vi "100kHz PID - Arbitration.vi"() -> ()   [LabVIEW 2010]
uses:
  <vilib>/eio/EIONode/EIONode.xnode
  <vilib>/rvi/eio/nirviEIOImplementation/nirviEIOImplementation.xnode
  <vilib>/rvi/eio/common/nirviEmuClasses.ctl
  <vilib>/addons/control/pid/fpga.llb/XNode/niFpgaPID.xnode
  <vilib>/rvi/eio/common/nirviEmuTemplateMethod_noerrors.vi
panel:
  in  "PID.Setpoint.PID 3":i16
  in  "PID.Proportional Gain.PID 3":i16=1
  in  "PID.Integral Gain.PID 3":i16
  in  "PID.Derivative Gain.PID 3":i16
  out "PID.Num Ticks 3":u32
  in  "PID.Setpoint.PID 2":i16
  in  "PID.Proportional Gain.PID 2":i16=1
  in  "PID.Integral Gain.PID 2":i16
  in  "PID.Derivative Gain.PID 2":i16
  out "PID.Num Ticks2":u32
  out "PID.Num Ticks 1":u32
  out "PID.Num Ticks":u32
  in  "PID.Setpoint.PID 1":i16
  in  "PID.Proportional Gain.PID 1":i16=1
  in  "PID.Integral Gain.PID 1":i16
  in  "PID.Derivative Gain.PID 1":i16
  in  "PID.Setpoint.PID 0":i16
  in  "PID.Proportional Gain.PID 0":i16=1
  in  "PID.Integral Gain.PID 0":i16
  in  "PID.Derivative Gain.PID 0":i16
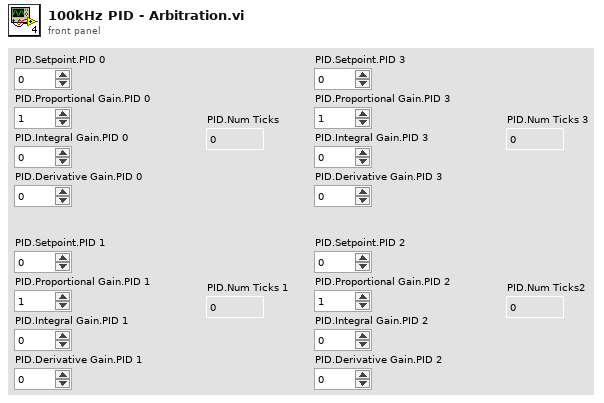
[diagram p1: front panel]
types:
  T1 = cluster{"proportional gain (Kc)":i16, "integral gain (Kc*Ts/Ti)":i16, "derivative gain (Kc*Td/Ts)":i16}
  T2 = typedef "nirviEmuClasses.ctl" = enum16{"IO Read", "IO Write", "Method", "Property Read", "Property Write"}
  T3 = cluster{"proportional gain (Kc)":fxp<+/-,16,8>, "proportional gain (Kc)":fxp<+/-,16,8>, "proportional gain (Kc)":fxp<+/-,16,8>}
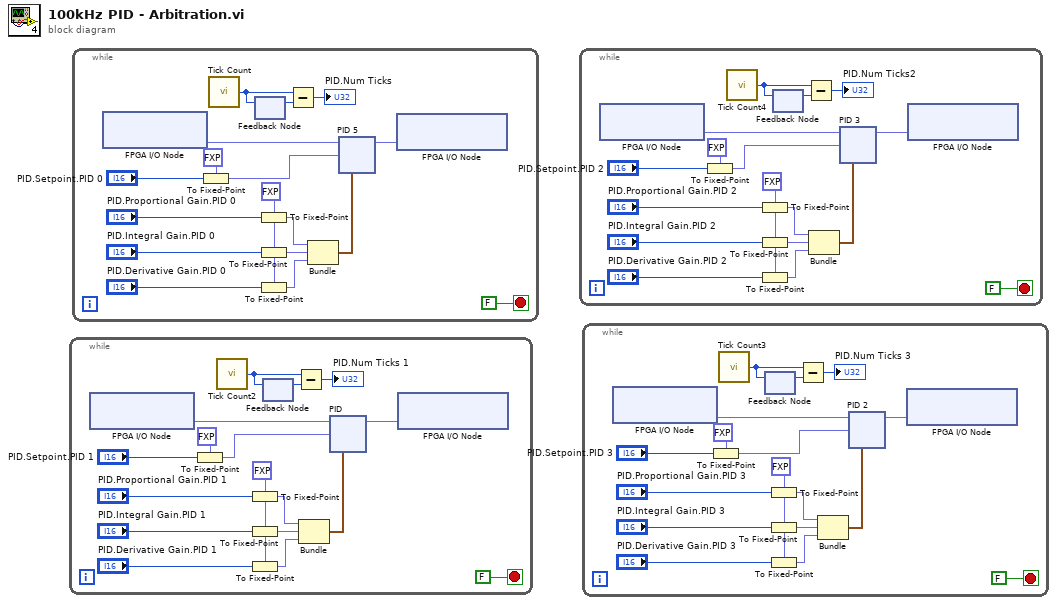
[diagram p0: block diagram]
diagram:
  n1 = while {
    stop <- FALSE stop-if-true
    w10 = fxp<+/-,16,8> 0.0 ("proportional gain (Kc)")
    n2 = xnode "FPGA I/O Node"() -> ("NI 9215/AI1"=w6:fxp<+/-,20,5>)  [unwired: 1 in, 1 out]
    n3 = To Fixed-Point(fixed-point type=fxp<+/-,16,5> 0.0 ("setpoint"), number="PID.Setpoint.PID 1") -> (fixed-point=w8:fxp<+/-,16,5>)
    n4 = call "Tick Count2"() -> ("Tick Count(Ticks)"=w2:u32)
    n5 = To Fixed-Point(fixed-point type=w10, number="PID.Proportional Gain.PID 1") -> (fixed-point=w13:fxp<+/-,16,8>)
    n6 = To Fixed-Point(fixed-point type=w10, number="PID.Integral Gain.PID 1") -> (fixed-point=w12:fxp<+/-,16,8>)
    n7 = To Fixed-Point(fixed-point type=w10, number="PID.Derivative Gain.PID 1") -> (fixed-point=w11:fxp<+/-,16,8>)
    n8 = feedback #1() -> (w1:u32)  [unwired: 1 in]
    n9 = feedback-in #1(w2) -> ()
    n10 = Subtract(x=w2, y=w1) -> (x-y=→"PID.Num Ticks 1":u32)
    n11 = Bundle("proportional gain (Kc)"=w13, "proportional gain (Kc)"=w12, "proportional gain (Kc)"=w11) -> (w14:T3)  [unwired: 1 in]
    n12 = xnode ("PID")("process variable"=w6, "setpoint"=w8, "PID gains"=w14) -> ("output"=w5:fxp<+/-,16,5>)  [unwired: 2 in]
    n13 = xnode "FPGA I/O Node"("NI 9263/AO1"=w5) -> ()  [unwired: 1 in, 1 out]
  }
  n14 = while {
    stop <- FALSE stop-if-true
    w92 = fxp<+/-,16,8> 0.0 ("proportional gain (Kc)")
    n15 = xnode "FPGA I/O Node"() -> ("NI 9215/AI0"=w100:fxp<+/-,20,5>)  [unwired: 1 in, 1 out]
    n16 = To Fixed-Point(fixed-point type=fxp<+/-,16,5> 0.0 ("setpoint"), number="PID.Setpoint.PID 0") -> (fixed-point=w88:fxp<+/-,16,5>)
    n17 = call "Tick Count"() -> ("Tick Count(Ticks)"=w85:u32)
    n18 = feedback #2() -> (w86:u32)  [unwired: 1 in]
    n19 = feedback-in #2(w85) -> ()
    n20 = To Fixed-Point(fixed-point type=w92, number="PID.Proportional Gain.PID 0") -> (fixed-point=w95:fxp<+/-,16,8>)
    n21 = To Fixed-Point(fixed-point type=w92, number="PID.Integral Gain.PID 0") -> (fixed-point=w94:fxp<+/-,16,8>)
    n22 = To Fixed-Point(fixed-point type=w92, number="PID.Derivative Gain.PID 0") -> (fixed-point=w93:fxp<+/-,16,8>)
    n23 = Subtract(x=w85, y=w86) -> (x-y=→"PID.Num Ticks":u32)
    n24 = Bundle("proportional gain (Kc)"=w95, "proportional gain (Kc)"=w94, "proportional gain (Kc)"=w93) -> (w96:T3)  [unwired: 1 in]
    n25 = xnode ("PID 5")("process variable"=w100, "setpoint"=w88, "PID gains"=w96) -> ("output"=w87:fxp<+/-,16,5>)  [unwired: 2 in]
    n26 = xnode "FPGA I/O Node"("NI 9263/AO0"=w87) -> ()  [unwired: 1 in, 1 out]
  }
  n27 = while {
    stop <- FALSE stop-if-true
    w176 = fxp<+/-,16,8> 0.0 ("proportional gain (Kc)")
    n28 = xnode "FPGA I/O Node"() -> ("NI 9215/AI2"=w172:fxp<+/-,20,5>)  [unwired: 1 in, 1 out]
    n29 = To Fixed-Point(fixed-point type=fxp<+/-,16,5> 0.0 ("setpoint"), number="PID.Setpoint.PID 2") -> (fixed-point=w174:fxp<+/-,16,5>)
    n30 = call "Tick Count4"() -> ("Tick Count(Ticks)"=w168:u32)
    n31 = To Fixed-Point(fixed-point type=w176, number="PID.Proportional Gain.PID 2") -> (fixed-point=w179:fxp<+/-,16,8>)
    n32 = To Fixed-Point(fixed-point type=w176, number="PID.Integral Gain.PID 2") -> (fixed-point=w178:fxp<+/-,16,8>)
    n33 = To Fixed-Point(fixed-point type=w176, number="PID.Derivative Gain.PID 2") -> (fixed-point=w177:fxp<+/-,16,8>)
    n34 = feedback #3() -> (w167:u32)  [unwired: 1 in]
    n35 = feedback-in #3(w168) -> ()
    n36 = Subtract(x=w168, y=w167) -> (x-y=→"PID.Num Ticks2":u32)
    n37 = Bundle("proportional gain (Kc)"=w179, "proportional gain (Kc)"=w178, "proportional gain (Kc)"=w177) -> (w180:T3)  [unwired: 1 in]
    n38 = xnode ("PID 3")("process variable"=w172, "setpoint"=w174, "PID gains"=w180) -> ("output"=w171:fxp<+/-,16,5>)  [unwired: 2 in]
    n39 = xnode "FPGA I/O Node"("NI 9263/AO2"=w171) -> ()  [unwired: 1 in, 1 out]
  }
  n40 = while {
    stop <- FALSE stop-if-true
    w258 = fxp<+/-,16,8> 0.0 ("proportional gain (Kc)")
    n41 = xnode "FPGA I/O Node"() -> ("NI 9215/AI3"=w266:fxp<+/-,20,5>)  [unwired: 1 in, 1 out]
    n42 = To Fixed-Point(fixed-point type=fxp<+/-,16,5> 0.0 ("setpoint"), number="PID.Setpoint.PID 3") -> (fixed-point=w254:fxp<+/-,16,5>)
    n43 = call "Tick Count3"() -> ("Tick Count(Ticks)"=w251:u32)
    n44 = feedback #4() -> (w252:u32)  [unwired: 1 in]
    n45 = feedback-in #4(w251) -> ()
    n46 = To Fixed-Point(fixed-point type=w258, number="PID.Proportional Gain.PID 3") -> (fixed-point=w261:fxp<+/-,16,8>)
    n47 = To Fixed-Point(fixed-point type=w258, number="PID.Integral Gain.PID 3") -> (fixed-point=w260:fxp<+/-,16,8>)
    n48 = To Fixed-Point(fixed-point type=w258, number="PID.Derivative Gain.PID 3") -> (fixed-point=w259:fxp<+/-,16,8>)
    n49 = Subtract(x=w251, y=w252) -> (x-y=→"PID.Num Ticks 3":u32)
    n50 = Bundle("proportional gain (Kc)"=w261, "proportional gain (Kc)"=w260, "proportional gain (Kc)"=w259) -> (w262:T3)  [unwired: 1 in]
    n51 = xnode ("PID 2")("process variable"=w266, "setpoint"=w254, "PID gains"=w262) -> ("output"=w253:fxp<+/-,16,5>)  [unwired: 2 in]
    n52 = xnode "FPGA I/O Node"("NI 9263/AO3"=w253) -> ()  [unwired: 1 in, 1 out]
  }
